vi "Host.vi"() -> ()   [LabVIEW 2020]
uses:
  FPGA/Libraries/Raster/Triangle.ctl
  FPGA/Libraries/Raster/Vertex.ctl
  FPGA/Libraries/Raster/Vector 3D.ctl
  FPGA/Libraries/Raster/UV.ctl
  Libraries/Utility/Convert Pixels To Picture.vi/d601d993-a776-4dc8-89c7-357d8398c88c.vi
  Libraries/Utility/Convert Pixels To Picture.vi/7816d0d6-8e4d-41a2-85ac-ed82f1435763.vi
  <vilib>/Utility/High Resolution Relative Seconds.vi
  <vilib>/FPGAPlugInAG/PXI-7952R/niLvFpga_Open_PXI-7952R.vi
  <vilib>/FPGAPlugInAG/PXI-7952R/niLvFpga_Reset_PXI-7952R.vi
  <vilib>/Utility/error.llb/Error Cluster From Error Code.vi
  <vilib>/rvi/errors/niLvFpgaAdjustHostInterfaceError.vi
  <vilib>/FPGAPlugInAG/PXI-7952R/niLvFpga_Run_PXI-7952R.vi
  <vilib>/picture/picture.llb/Draw Unflattened Pixmap.vi
  <vilib>/picture/picture.llb/Draw True-Color Pixmap.vi
  <vilib>/rvi/interface/nirviOpenFPGA/nirviOpenFPGA.xnode
  Builds/FPGA/TestDRAM.lvbitx
  <vilib>/rvi/interface/nirviMethod/nirviMethod.xnode
  <vilib>/rvi/interface/nirviReadWriteControl/nirviReadWriteControl.xnode
  <vilib>/rvi/errors/niLvFpgaMergeErrorWithErrorCode.vi
  <vilib>/FPGAPlugInAG/PXI-7952R/niLvFpga_ReadFifo_PXI-7952R.vi
  NiFpgaLv.dll
  FPGA/Libraries/Raster/Raster (FPGA).lvlib
  Libraries/Utility/Utility.lvlib
  <vilib>/FPGAPlugInAG/PXI-7952R/niLvFpga_ConfigureFifo_PXI-7952R.vi
  <vilib>/FPGAPlugInAG/PXI-7952R/niLvFpga_StartFifo_PXI-7952R.vi
panel:
  in  "Raster Loop Wait [ticks]":u32=1000000
  out "2D Picture":picture
  out "output array":u32[](array[numeric])
  in  "Send To Host":bool
  out "Latest Data":cluster{"Address":i32, "Value":u32}
  out "Numeric":u32
  out "Waveform Graph":u32[](graph)
  out "Data 2":u32[](array[numeric])
  out "Actual Depth":u32
  out "DRAM Read Address":u32
  out "To DRAM Timed Out?":bool
  out "Raster Loop Index":i32
  out "Data":u32[](array[numeric])
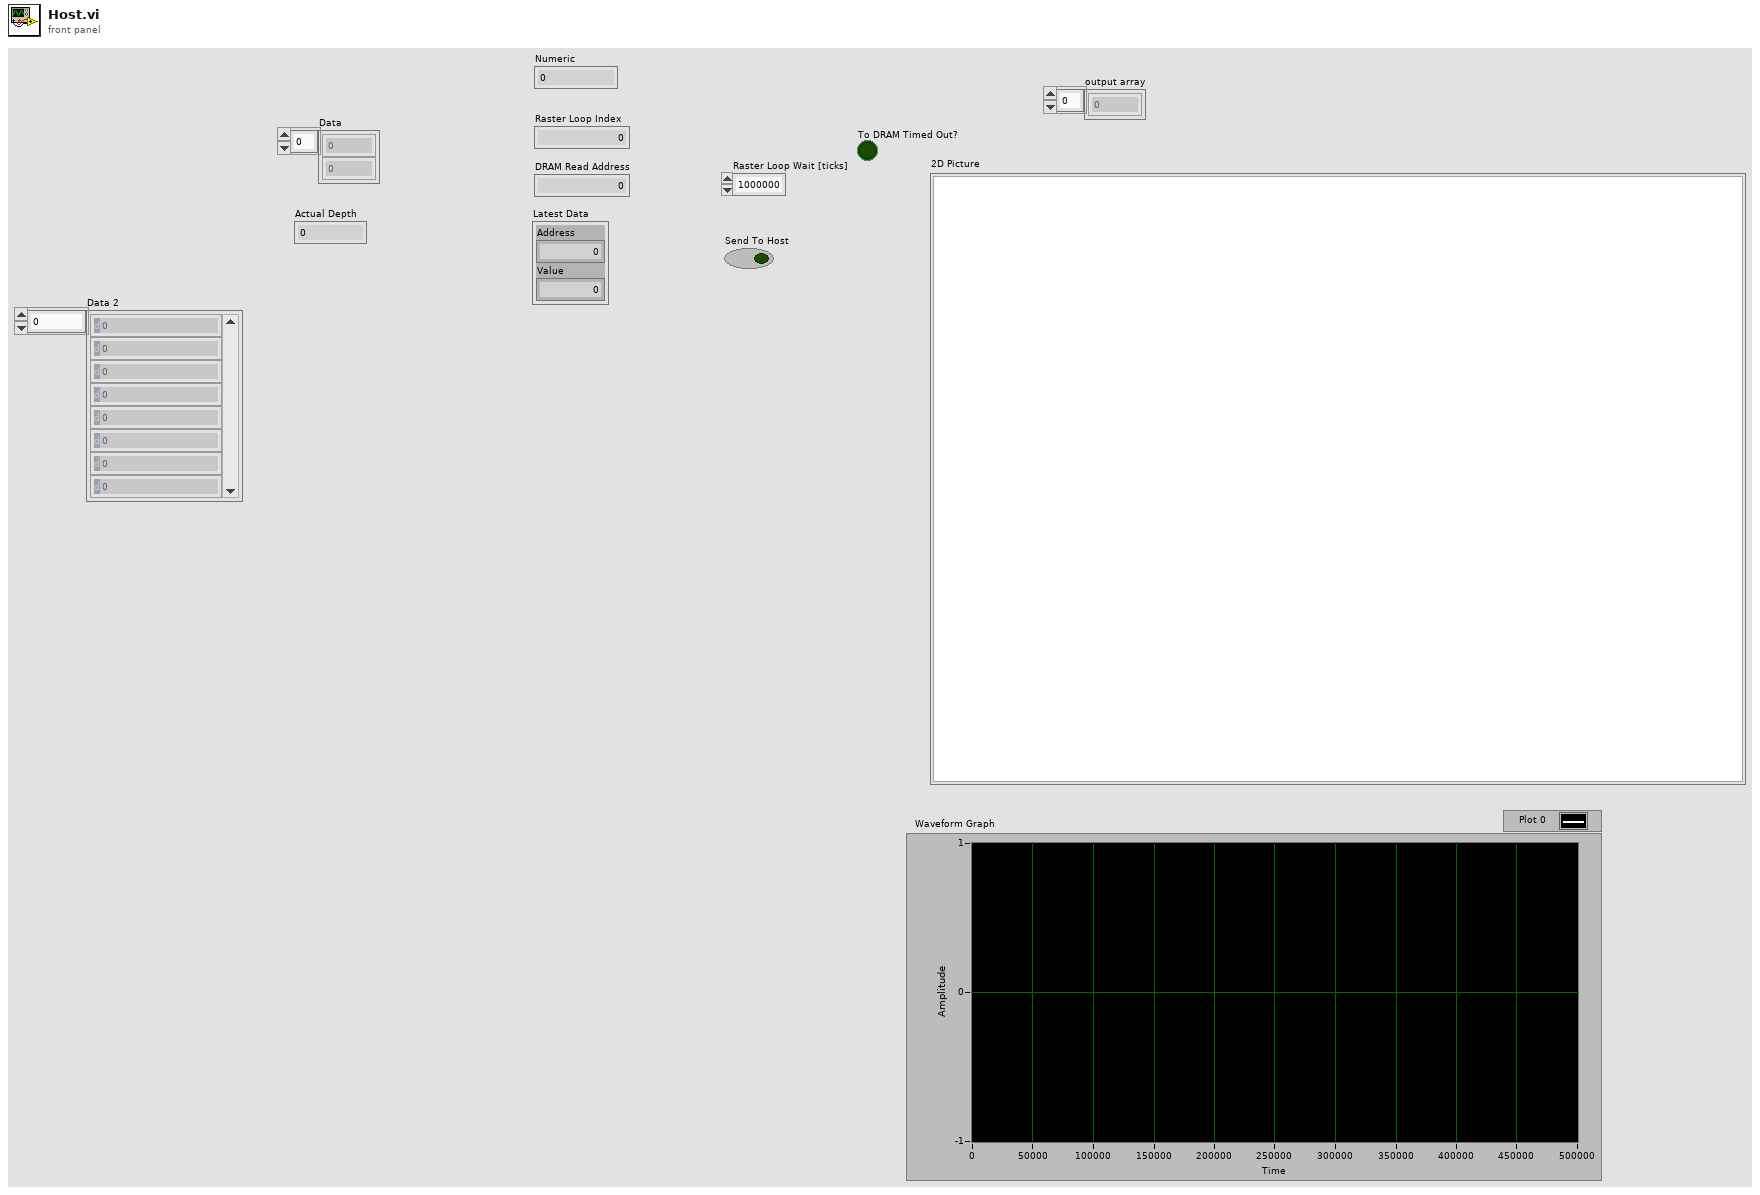
[diagram p1: front panel]
types:
  T1 = typedef "Raster (FPGA).lvlib/Triangle.ctl" = cluster{"Vertex 1":T2, "Vertex 2":T2, "Vertex 3":T2, "Colour":u32}
  T2 = typedef "Raster (FPGA).lvlib/Vertex.ctl" = cluster{"Position":T3, "UV":T4, "Colour":u32}
  T3 = typedef "Raster (FPGA).lvlib/Vector 3D.ctl" = cluster{"x":sgl, "y":sgl, "z":sgl}
  T4 = typedef "Raster (FPGA).lvlib/UV.ctl" = cluster{"u":sgl, "v":sgl}
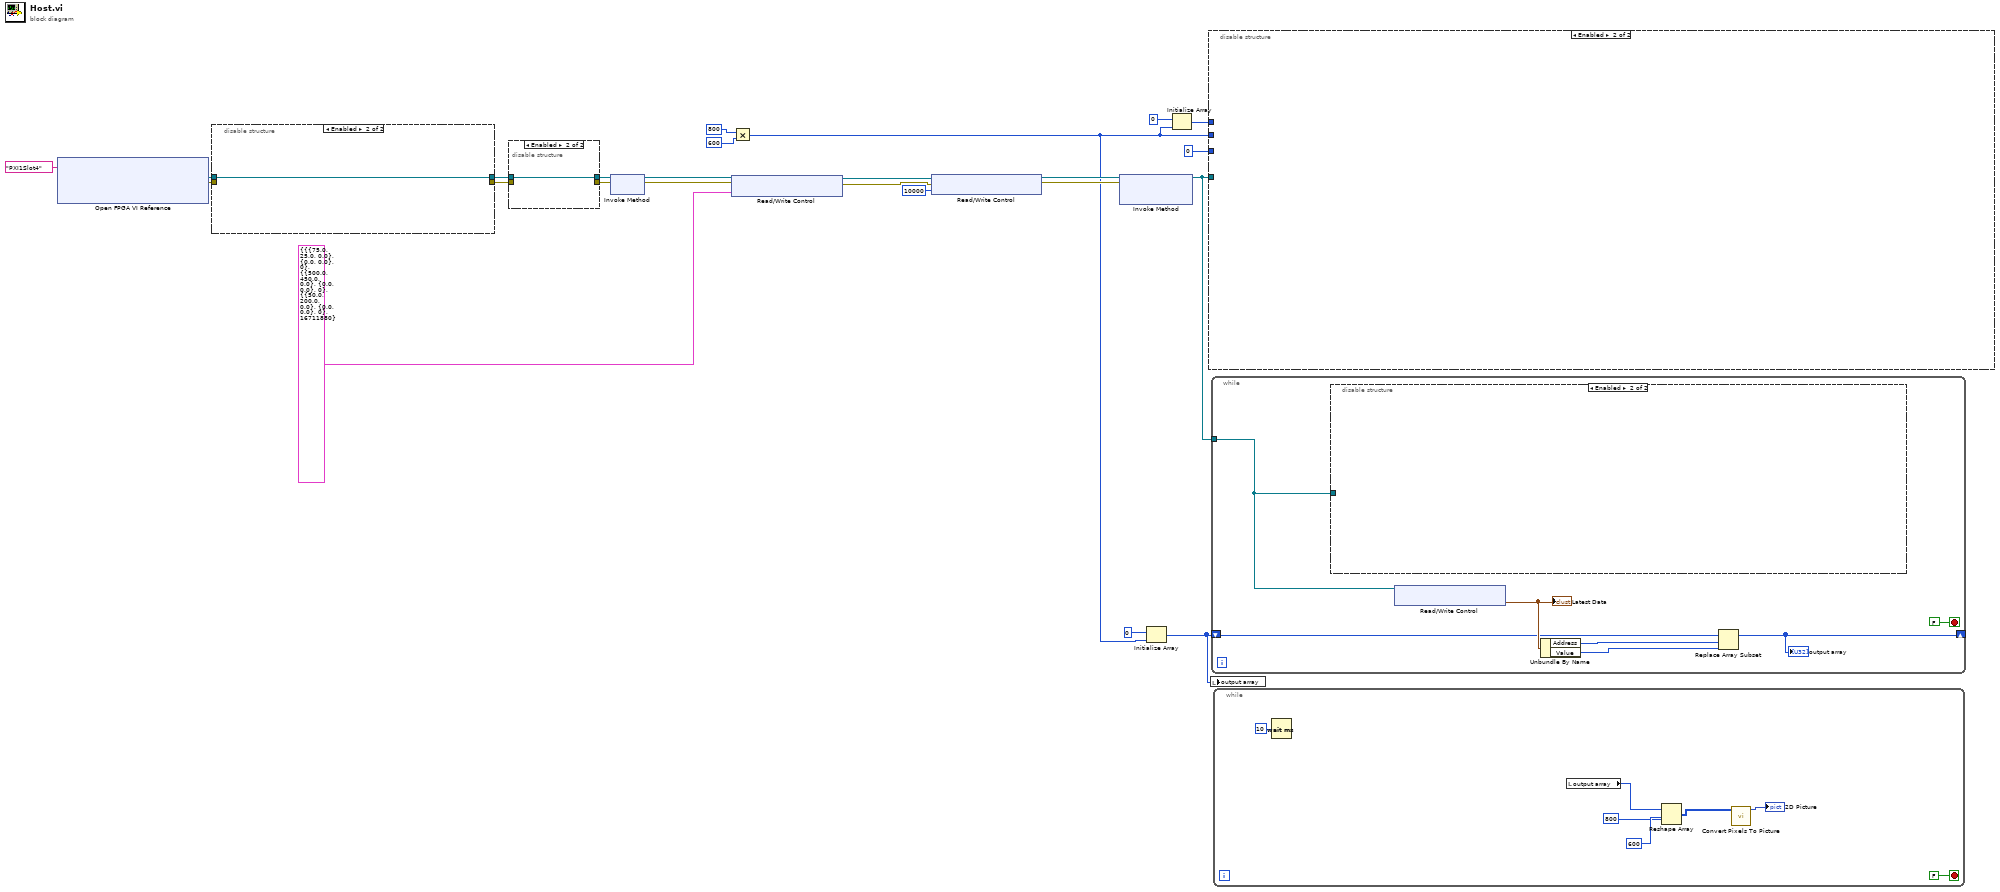
[diagram p0: block diagram]
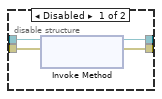
[diagram p2: hidden frame]
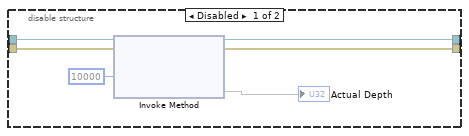
[diagram p3: hidden frame]
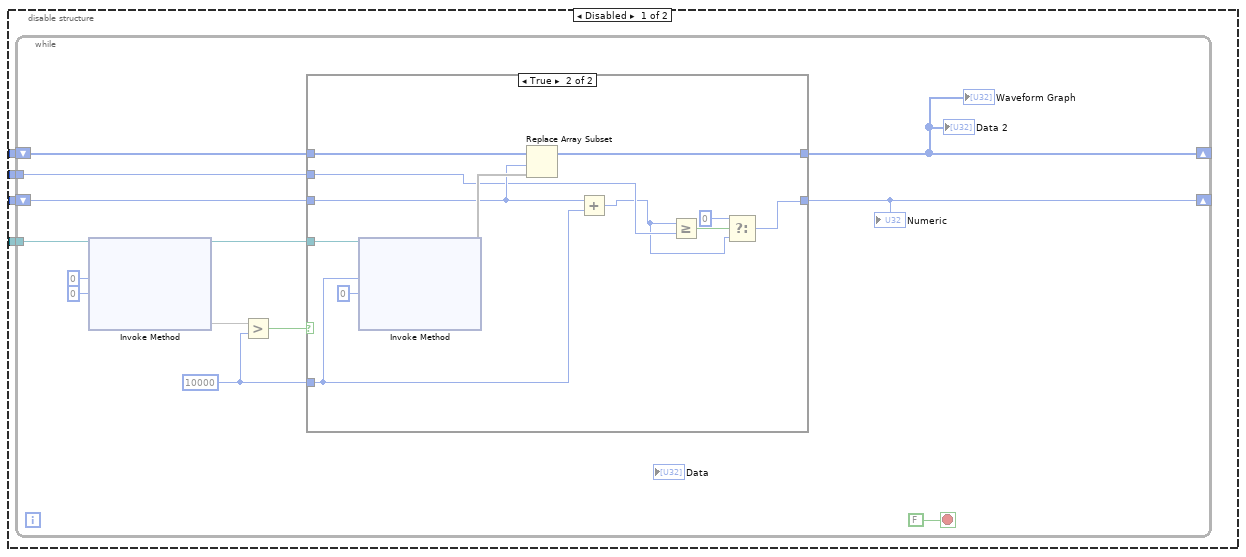
[diagram p4: hidden frame]
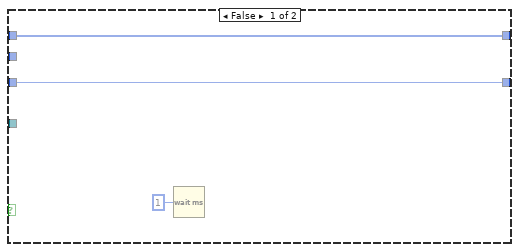
[diagram p5: hidden frame]
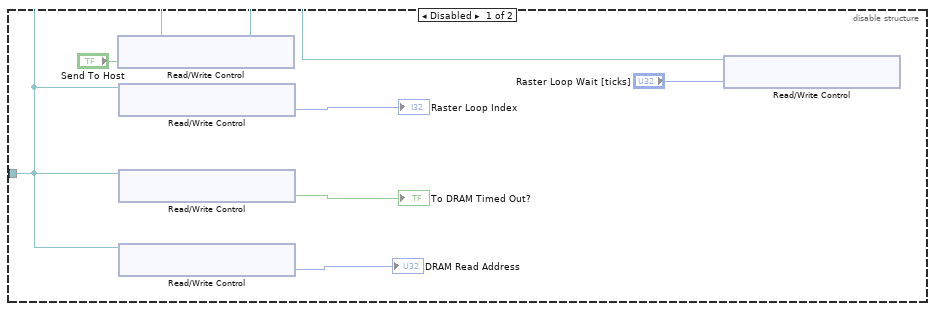
[diagram p6: hidden frame]
diagram:
  n1 = xnode "Open FPGA VI Reference"("resource name"=tag "PXI1Slot4") -> ("FPGA VI Reference Out"=w21:refnum<k20>, "error out"=w20:errorcluster)  [unwired: 1 in]
  n2 = disable-structure shown="Enabled" {
    disable-tunnel: w21 -> [w30 w31]
    disable-tunnel: w20 -> [w29 _]
    disable-tunnel: [w26 _] -> w7
    disable-tunnel: [w25 w31] -> w6
    frame Disabled {
      n3 = xnode "Invoke Method"("FPGA VI Reference In"=w30, "error in"=w29, "Requested Depth"=u32 10000) -> ("FPGA VI Reference Out"=w25:refnum<k20>, "error out"=w26:errorcluster, "Actual Depth"=→"Actual Depth")
    }
    frame Enabled {
    }
  }
  n4 = disable-structure shown="Enabled" {
    disable-tunnel: [w35 w36] -> w23
    disable-tunnel: [w34 _] -> w22
    disable-tunnel: w7 -> [w33 _]
    disable-tunnel: w6 -> [w32 w36]
    frame Disabled {
      n5 = xnode "Invoke Method"("FPGA VI Reference In"=w32, "error in"=w33) -> ("FPGA VI Reference Out"=w35:refnum<k20>, "error out"=w34:errorcluster)
    }
    frame Enabled {
    }
  }
  n6 = xnode "Invoke Method"("FPGA VI Reference In"=w23, "error in"=w22) -> ("FPGA VI Reference Out"=w5:refnum<k20>, "error out"=w4:errorcluster)
  n7 = xnode "Read/Write Control"("FPGA VI Reference In"=w5, "error in"=w4, "Triangle"=T1 {"Vertex 1"={"Position"={"x"=75.0, "y"=25.0, "z"=0.0}, "UV"={"u"=0.0, "v"=0.0}, "Colour"=0}, "Vertex 2"={"Position"={"x"=500.0, "y"=450.0, "z"=0.0}, "UV"={"u"=0.0, "v"=0.0}, "Colour"=0}, "Vertex 3"={"Position"={"x"=50.0, "y"=200.0, "z"=0.0}, "UV"={"u"=0.0, "v"=0.0}, "Colour"=0}, "Colour"=16711880}) -> ("FPGA VI Reference Out"=w2:refnum<k20>, "error out"=w3:errorcluster)
  n8 = Multiply(x=u32 800, y=u32 600) -> (x*y=w8:u32)
  n9 = xnode "Read/Write Control"("FPGA VI Reference In"=w2, "error in"=w3, "Raster Loop Wait [ticks]"=u32 10000) -> ("FPGA VI Reference Out"=w11:refnum<k20>, "error out"=w10:errorcluster)
  n10 = xnode "Invoke Method"("FPGA VI Reference In"=w11, "error in"=w10) -> ("FPGA VI Reference Out"=w19:refnum<k20>)  [unwired: 1 in, 1 out]
  n11 = Initialize Array(u32 0, w8) -> (w1:u32[])
  n12 = Initialize Array(u32 0, w8) -> (w18:u32[])
  n13 = disable-structure shown="Enabled" {
    disable-tunnel: w19 -> [w40 _]
    disable-tunnel: w18 -> [w39 _]
    disable-tunnel: 0 -> [w38 _]
    disable-tunnel: w8 -> [w37 _]
    frame Disabled {
      n14 = while {
        tunnel: w40 -> [w53]
        shift-right: [w43] -> _
        shift-left: w39 -> [w46]
        shift-right: [w44] -> _
        shift-left: w38 -> [w45]
        tunnel: w37 -> [w41]
        stop <- FALSE stop-if-true
        w48 = u32 10000 ("y")
        n15 = xnode "Invoke Method"("FPGA VI Reference In"=w53, "Number of Elements"=u32 0, "Timeout (ms)"=0) -> ("FPGA VI Reference Out"=w47:refnum<k20>, "Elements Remaining"=w50)  [unwired: 1 in, 2 out]
        n16 = Greater?(x=w50, y=w48) -> (0:w49:bool)
        n17 = case shown="True" w49 {
          tunnel: w48 -> [_ w63]
          tunnel: w47 -> [_ w67]
          tunnel: w46 -> [w56 w66]
          tunnel: [w56 w64] -> w43
          tunnel: w45 -> [w55 w62]
          tunnel: [w55 w57] -> w44
          tunnel: w41 -> [_ w61]
          frame False {
            n18 = Wait (ms)(milliseconds to wait=u32 1) -> ()  [unwired: 1 out]
          }
          frame True {
            n19 = xnode "Invoke Method"("FPGA VI Reference In"=w67, "Number of Elements"=w63, "Timeout (ms)"=0) -> ("Data"=w65:void[])  [unwired: 1 in, 3 out]
            n20 = Replace Array Subset(array=w66, new element=w65, index=w62) -> (w64:u32[])
            n21 = Add(x=w62, y=w63) -> (x+y=w58:u32)
            n22 = Greater Or Equal?(x=w58, y=w61) -> (x >= y?=w60:bool)
            n23 = Select(t=u32 0, s=w60, f=w58) -> (s? t:f=w57:u32)
          }
        }
        "Data 2" <- w43
        "Waveform Graph" <- w43
        "Numeric" <- w44
      }
    }
    frame Enabled {
    }
  }
  n24 = local write "output array"(w1) -> ()
  n25 = while {
    tunnel: w19 -> [w74]
    shift-right: [w69] -> _
    shift-left: w1 -> [w72]
    stop <- FALSE stop-if-true
    n26 = disable-structure shown="Enabled" {
      disable-tunnel: w74 -> [w82 _]
      frame Disabled {
        n27 = xnode "Read/Write Control"("FPGA VI Reference In"=w82, "Send To Host"="Send To Host") -> ("FPGA VI Reference Out"=w76:refnum<k20>)  [unwired: 1 in, 1 out]
        n28 = xnode "Read/Write Control"("FPGA VI Reference In"=w82) -> ("Raster Loop Index"=→"Raster Loop Index":i32)  [unwired: 1 in, 2 out]
        n29 = xnode "Read/Write Control"("FPGA VI Reference In"=w82) -> ("To DRAM Timed Out?"=→"To DRAM Timed Out?":bool)  [unwired: 1 in, 2 out]
        n30 = xnode "Read/Write Control"("FPGA VI Reference In"=w82) -> ("DRAM Read Address"=→"DRAM Read Address":u32)  [unwired: 1 in, 2 out]
        n31 = xnode "Read/Write Control"("FPGA VI Reference In"=w76, "Raster Loop Wait [ticks]"="Raster Loop Wait [ticks]") -> ()  [unwired: 1 in, 2 out]
      }
      frame Enabled {
      }
    }
    n32 = xnode "Read/Write Control"("FPGA VI Reference In"=w74) -> ("Latest Data"=w73:cluster{"Address":i32, "Value":u32})  [unwired: 1 in, 2 out]
    "Latest Data" <- w73
    n33 = Unbundle By Name(w73) -> ("Address"=w71:i32, "Value"=w70:u32)
    n34 = Replace Array Subset(array=w72, new element=w70, index=w71) -> (w69:u32[])
    "output array" <- w69
  }
  n35 = while {
    stop <- FALSE stop-if-true
    n36 = Wait (ms)(milliseconds to wait=u32 10) -> ()  [unwired: 1 out]
    n37 = local read "output array"() -> (w89:u32[])
    n38 = Reshape Array(w89, 600 ("dimension size"), 800 ("dimension size")) -> (w88:u32[][])
    n39 = call "Convert Pixels To Picture.vi"("Pixel Data in"=w88) -> ("2D Picture"=→"2D Picture":picture)  [unwired: 9 in, 1 out]
  }
